vi "State Control.vi"() -> ()   [LabVIEW 2020]
uses:
  TCP Comms/State.ctl
  TCP Comms/TinyTCP.lvlib
panel:
  in  "State":T1
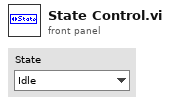
[diagram p1: front panel]
types:
  T1 = typedef "TinyTCP.lvlib/State.ctl" = enum16{"Idle", "Starting", "Connecting", "Connected", "Disconnecting", "Stopped"}
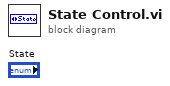
[diagram p0: block diagram]
diagram:
